vi "Create_PMT_Dir.vi"(0 "Test":string, 1 "Run":string, 3 "PMTs":string[](array[string])) -> (7 "Paths":path[](array[path]))   [LabVIEW 2018]
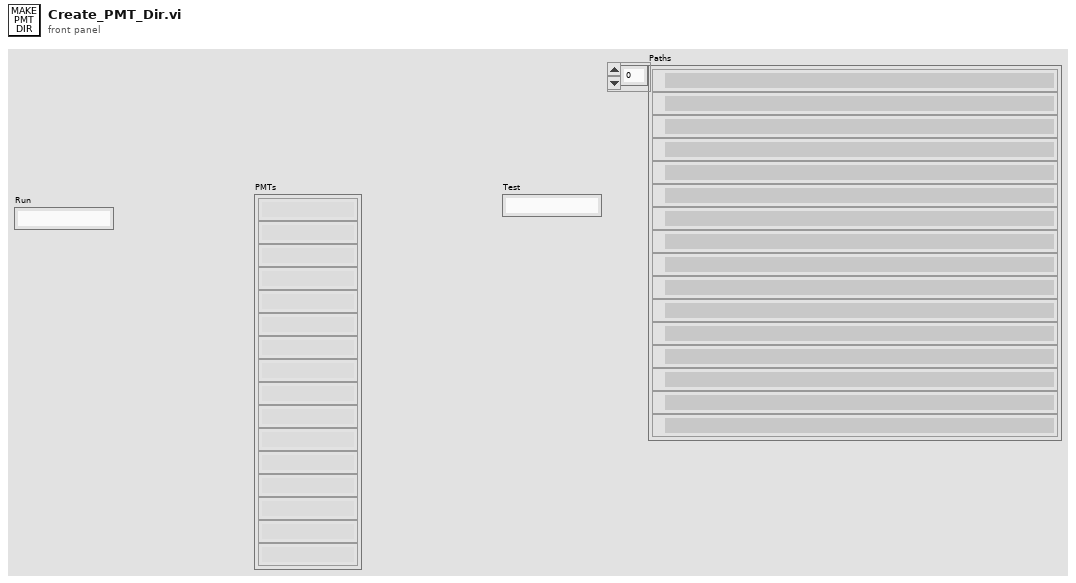
[diagram p1: front panel]
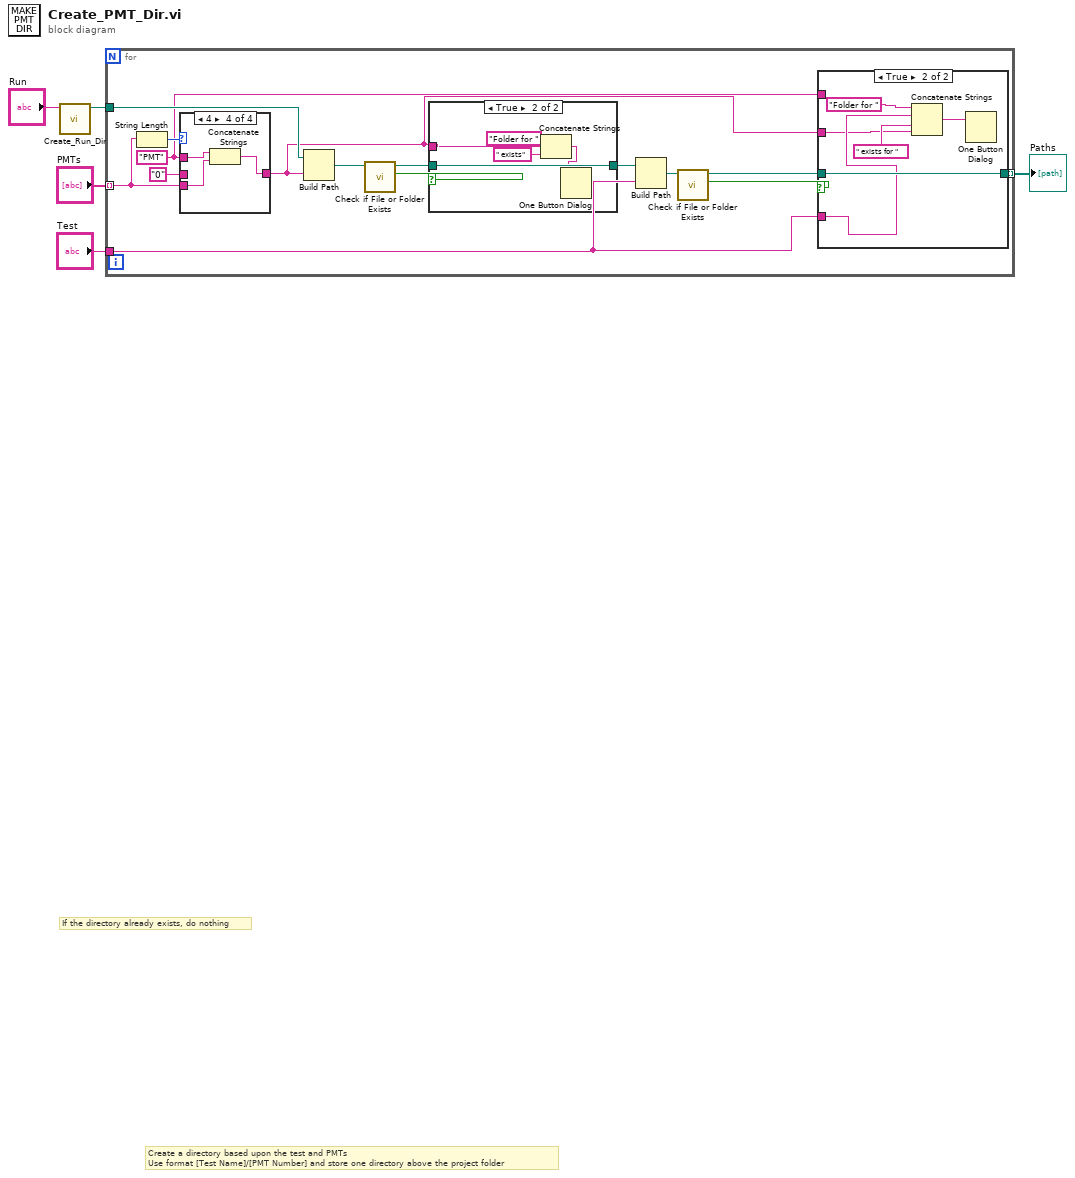
[diagram p0: block diagram]
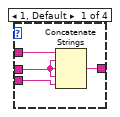
[diagram p2: hidden frame]
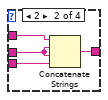
[diagram p3: hidden frame]
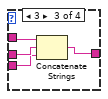
[diagram p4: hidden frame]
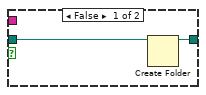
[diagram p5: hidden frame]
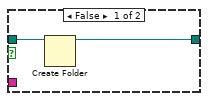
[diagram p6: hidden frame]
diagram:
  # "If the directory already exists, do nothing"
  # "Create a directory based upon the test and PMTs\nUse format [Test Name]/[PMT Number] and store one directory above the project folder"
  n1 = call "Create_Run_Dir.vi"("Run"="Run") -> ("dup path"=w2:path)  [unwired: 7 in, 3 out]
  n2 = for {
    tunnel: "PMTs" -> [w9] mode=indexing
    tunnel: w2 -> [w20]
    tunnel: "Test" -> [w7]
    tunnel: [w12] -> w1 mode=indexing
    w10 = "PMT" ("string")
    n3 = String Length(string=w9) -> (length=w11:i32)
    n4 = case shown="4" w11 {
      tunnel: w10 -> [w24 w27 w32 w35]
      tunnel: w9 -> [w22 w25 w30 w34]
      tunnel: [w23 w28 w29 w33] -> w6
      tunnel: "0" ("string") -> [w21 w26 w31 _]
      frame 1, Default {
        n5 = Concatenate Strings(w24, w21, w21, w21, w22) -> (w23:string)
      }
      frame 2 {
        n6 = Concatenate Strings(w27, w26, w26, w25) -> (w28:string)
      }
      frame 3 {
        n7 = Concatenate Strings(w32, w31, w30) -> (w29:string)
      }
      frame 4 {
        n8 = Concatenate Strings(w35, w34) -> (w33:string)
      }
    }
    n9 = Build Path(base path=w20, name or relative path=w6) -> (appended path=w16:path)
    n10 = call <vilib>:"Check if File or Folder Exists.vi"("path"=w16) -> ("file or folder exists?"=w15:bool, "dup path"=w14:path)  [unwired: 8 in, 1 out]
    n11 = case shown="True" w15 {
      tunnel: w14 -> [w37 w42]
      tunnel: [w36 w42] -> w13
      tunnel: w6 -> [_ w39]
      frame False {
        n12 = Create Folder(path (use dialog)=w37) -> (created path=w36:path)  [unwired: 2 in, 2 out]
      }
      frame True {
        n13 = Concatenate Strings("Folder for " ("string"), w39, " exists" ("string")) -> (w41:string)
        n14 = One Button Dialog(message=w41) -> ()  [unwired: 1 in, 1 out]
      }
    }
    n15 = Build Path(base path=w13, name or relative path=w7) -> (appended path=w19:path)
    n16 = call <vilib>:"Check if File or Folder Exists.vi"("path"=w19) -> ("file or folder exists?"=w18:bool, "dup path"=w17:path)  [unwired: 8 in, 1 out]
    n17 = case shown="True" w18 {
      tunnel: w17 -> [w44 w50]
      tunnel: [w43 w50] -> w12
      tunnel: w7 -> [_ w48]
      tunnel: w10 -> [_ _]
      tunnel: w6 -> [_ w46]
      frame False {
        n18 = Create Folder(path (use dialog)=w44) -> (created path=w43:path)  [unwired: 2 in, 2 out]
      }
      frame True {
        n19 = Concatenate Strings("Folder for " ("string"), w48, " exists for " ("string"), w46) -> (w45:string)
        n20 = One Button Dialog(message=w45) -> ()  [unwired: 1 in, 1 out]
      }
    }
  }
  "Paths" <- w1
